vi "ControlQuery.vi"(8 "error in (no error)":errorcluster, 11 "Cryostat in":refnum<class "Cryostat.lvclass">) -> (0 "error out":errorcluster, 3 "Cryostat out":refnum<class "Cryostat.lvclass">)   [LabVIEW 2017, in "Cryostat.lvclass"]
uses:
  Cryostat.lvclass
  Cryostat.lvclass/Cryostat.ctl
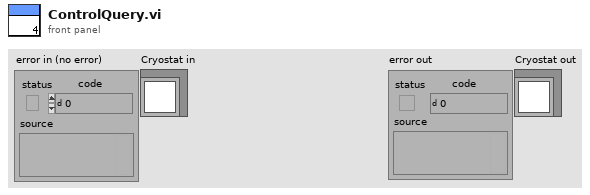
[diagram p1: front panel]
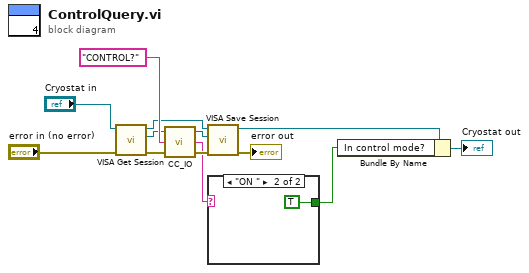
[diagram p0: block diagram]
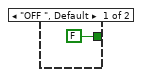
[diagram p2: hidden frame]
diagram:
  n1 = call-dynamic "VISA Get Session.vi"("error in (no error)"="error in (no error)", "Instrument.lvclass in"="Cryostat in") -> ("error out"=w11:errorcluster, "VISA Resource Name"=w7:refnum<visa-resource-name>, "Instrument.lvclass out"=w8:refnum<class "Cryostat.lvclass">)  [unwired: 7 out]
  n2 = call "CC_IO.vi"("error in (no error)"=w11, "Output Command"="CONTROL?", "VISA In"=w7) -> ("error out"=w12:errorcluster, "Input String"=w10:string, "VISA out"=w6:refnum<visa-resource-name>)
  n3 = call-dynamic "VISA Save Session.vi"("error in (no error)"=w12, "VISA Resource Name"=w6, "Instrument.lvclass in"=w8) -> ("error out"=→"error out":errorcluster, "Instrument.lvclass out"=w5:refnum<class "Cryostat.lvclass">)  [unwired: 7 out]
  n4 = case shown="\"ON \"" w10 {
    tunnel: [FALSE TRUE] -> w13
    frame "OFF ", Default {
    }
    frame "ON " {
    }
  }
  n5 = Bundle By Name(cluster=w5, "In control mode?"=w13) -> (→"Cryostat out":refnum<class "Cryostat.lvclass">)
